vi "Configure SequenceFileView Manager.vi"(8 "error in (no error)":errorcluster, 11 "Auto UI in":refnum<class "Auto UI.lvclass">) -> (0 "error out":errorcluster, 3 "Auto UI out":refnum<class "Auto UI.lvclass">)   [LabVIEW 2023, in "GUI.lvlib" / "Auto UI.lvlib" / "Auto UI.lvclass"]
uses:
  Auto UI.lvclass
  Auto UI.lvclass/Auto UI.ctl
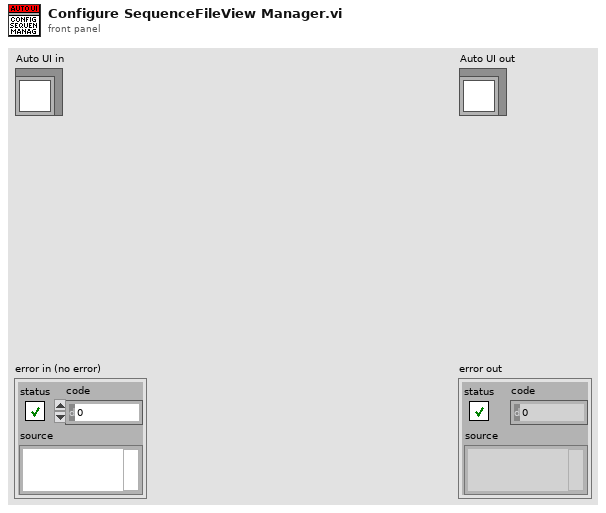
[diagram p1: front panel]
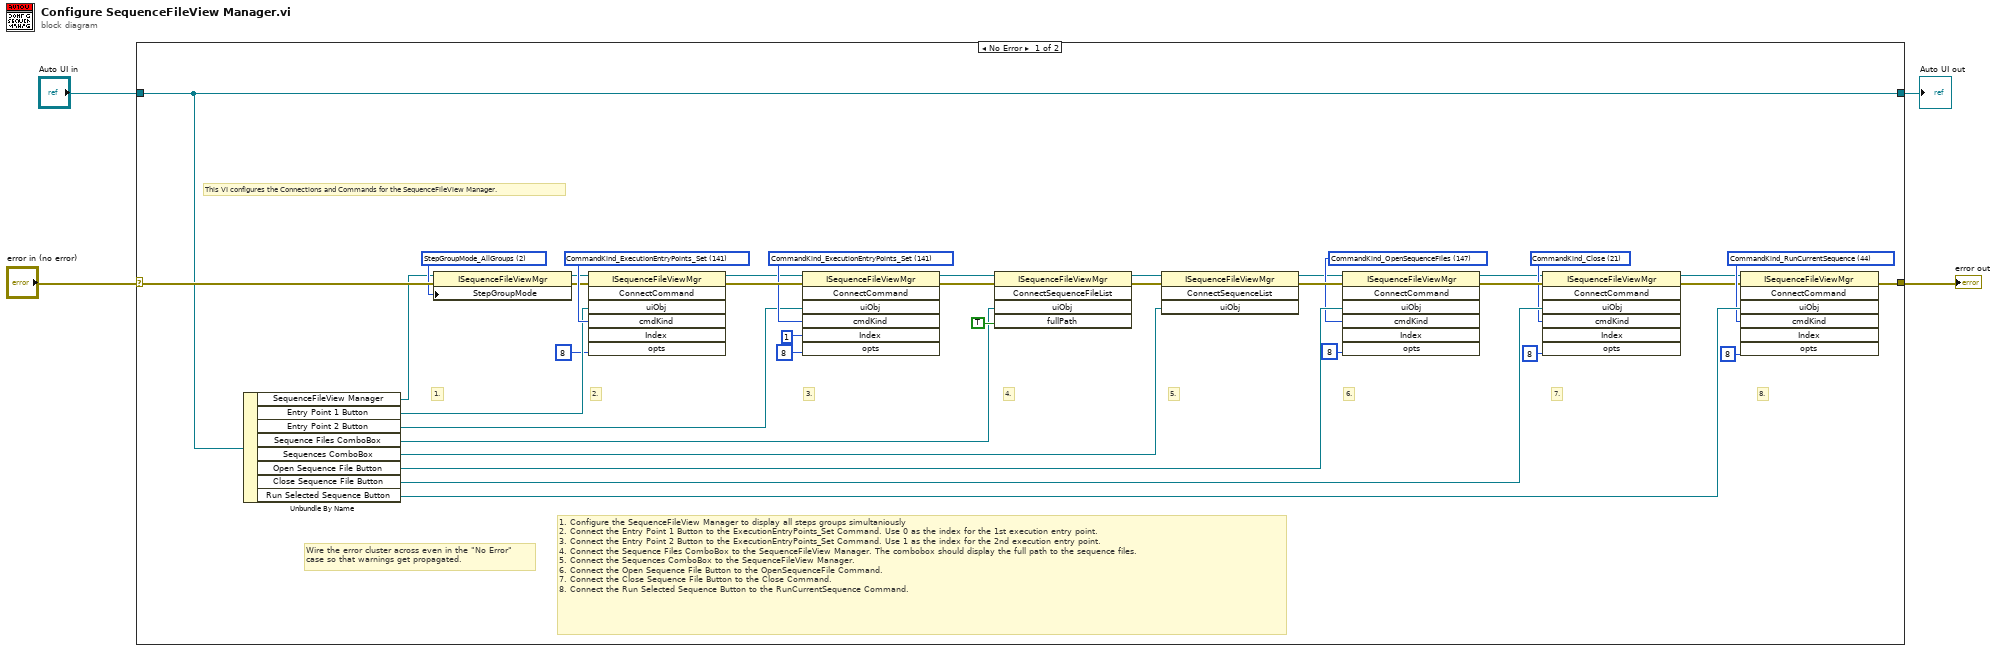
[diagram p0: block diagram]
diagram:
  n1 = case shown="No Error" "error in (no error)" {
    selector: "error in (no error)" -> [w42 w44]
    tunnel: [w41 w44] -> w3
    tunnel: [w5 w43] -> w1
    tunnel: "Auto UI in" -> [w5 w43]
    frame No Error {
      w24 = 2 items=["StepGroupMode_OneGroup"=1, "StepGroupMode_AllGroups"=2] ("StepGroupMode")
      w25 = 147 items=["CommandKind_NotACommand"=0, "CommandKind_Container"=1, "CommandKind_Separator"=2, "CommandKind_Custom"=3, "CommandKind_OpenSequenceFile"=20, "CommandKind_Close"=21, "CommandKind_CloseAll"=22, "CommandKind_CloseCompletedExecutions"=23, "CommandKind_OpenWorkspaceBrowser"=24, "CommandKind_Login"=25, "CommandKind_Logout"=26, "CommandKind_LoginLogout"=27, "CommandKind_UnloadAllModules"=28, "CommandKind_MRUFile"=29, "CommandKind_Exit"=30, "CommandKind_Restart"=40, "CommandKind_RunEntryPoint"=41, "CommandKind_RunEntryPointOnSelectedSteps"=42, "CommandKind_LoopEntryPointOnSelectedSteps"=43, "CommandKind_RunCurrentSequence"=44, "CommandKind_RunSpecificSequence"=45, "CommandKind_RunSelectedSteps"=46, "CommandKind_RunSelectedStepsUsingEntryPointsSubmenu"=47, "CommandKind_LoopOnSelectedSteps"=48, "CommandKind_LoopOnSelectedStepsUsingEntryPointsSubmenu"=49, "CommandKind_BreakOnFirstStep"=50, "CommandKind_BreakOnStepFailure"=51, "CommandKind_BreakOnSequenceFailure"=52, "CommandKind_TracingEnabled"=53, "CommandKind_ToggleBreakpoint"=60, "CommandKind_SetRunModeSubmenu"=61, "CommandKind_RunModeForcePass"=62, "CommandKind_RunModeForceFail"=63, "CommandKind_RunModeSkip"=64, "CommandKind_RunModeNormal"=65, "CommandKind_Resume"=66, "CommandKind_StepInto"=67, "CommandKind_StepOver"=68, "CommandKind_StepOut"=69, "CommandKind_SetNextStep"=70, "CommandKind_Break"=71, "CommandKind_BreakResume"=72, "CommandKind_Terminate"=73, "CommandKind_TerminateRestart"=74, "CommandKind_Abort"=75, "CommandKind_BreakAll"=76, "CommandKind_TerminateAll"=77, "CommandKind_AbortAll"=78, "CommandKind_ResumeAll"=79, "CommandKind_DisplayBreakpointsAndWatchExpressions"=80, "CommandKind_DisplayBreakpointSettings"=81, "CommandKind_BreakpointSubmenu"=85, "CommandKind_ConfigureAdapters"=90, "CommandKind_ConfigureStationOptions"=91, "CommandKind_ConfigureSearchDirectories"=92, "CommandKind_ConfigureExternalViewers"=93, "CommandKind_ToolItem"=100, "CommandKind_CustomizeTools"=101, "CommandKind_ExecutionEntryPointInsertionMarker"=110, "CommandKind_ExecutionEntryPointDefaultMenuInsertionMarker"=111, "CommandKind_ConfigurationEntryPointInsertionMarker"=112, "CommandKind_ConfigurationEntryPointDefaultMenuInsertionMarker"=113, "CommandKind_DefaultFileMenu_Set"=120, "CommandKind_DefaultExecuteMenu_Set"=121, "CommandKind_DefaultDebugMenu_Set"=123, "CommandKind_DefaultConfigureMenu_Set"=124, "CommandKind_DefaultToolsMenu_Set"=125, "CommandKind_DefaultSequenceViewContextMenu_Set"=126, "CommandKind_DefaultListBarContextMenu_Set"=127, "CommandKind_MRUFiles_Set"=140, "CommandKind_ExecutionEntryPoints_Set"=141, "CommandKind_RunSequences_Set"=142, "CommandKind_RunSelectedStepsUsingEntryPoints_Set"=143, "CommandKind_LoopOnSelectedStepsUsingEntryPoints_Set"=144, "CommandKind_ConfigurationEntryPoints_Set"=145, "CommandKind_Tools_Set"=146, "CommandKind_OpenSequenceFiles"=147] ("cmdKind")
      w26 = 44 items=["CommandKind_NotACommand"=0, "CommandKind_Container"=1, "CommandKind_Separator"=2, "CommandKind_Custom"=3, "CommandKind_OpenSequenceFile"=20, "CommandKind_Close"=21, "CommandKind_CloseAll"=22, "CommandKind_CloseCompletedExecutions"=23, "CommandKind_OpenWorkspaceBrowser"=24, "CommandKind_Login"=25, "CommandKind_Logout"=26, "CommandKind_LoginLogout"=27, "CommandKind_UnloadAllModules"=28, "CommandKind_MRUFile"=29, "CommandKind_Exit"=30, "CommandKind_Restart"=40, "CommandKind_RunEntryPoint"=41, "CommandKind_RunEntryPointOnSelectedSteps"=42, "CommandKind_LoopEntryPointOnSelectedSteps"=43, "CommandKind_RunCurrentSequence"=44, "CommandKind_RunSpecificSequence"=45, "CommandKind_RunSelectedSteps"=46, "CommandKind_RunSelectedStepsUsingEntryPointsSubmenu"=47, "CommandKind_LoopOnSelectedSteps"=48, "CommandKind_LoopOnSelectedStepsUsingEntryPointsSubmenu"=49, "CommandKind_BreakOnFirstStep"=50, "CommandKind_BreakOnStepFailure"=51, "CommandKind_BreakOnSequenceFailure"=52, "CommandKind_TracingEnabled"=53, "CommandKind_ToggleBreakpoint"=60, "CommandKind_SetRunModeSubmenu"=61, "CommandKind_RunModeForcePass"=62, "CommandKind_RunModeForceFail"=63, "CommandKind_RunModeSkip"=64, "CommandKind_RunModeNormal"=65, "CommandKind_Resume"=66, "CommandKind_StepInto"=67, "CommandKind_StepOver"=68, "CommandKind_StepOut"=69, "CommandKind_SetNextStep"=70, "CommandKind_Break"=71, "CommandKind_BreakResume"=72, "CommandKind_Terminate"=73, "CommandKind_TerminateRestart"=74, "CommandKind_Abort"=75, "CommandKind_BreakAll"=76, "CommandKind_TerminateAll"=77, "CommandKind_AbortAll"=78, "CommandKind_ResumeAll"=79, "CommandKind_DisplayBreakpointsAndWatchExpressions"=80, "CommandKind_DisplayBreakpointSettings"=81, "CommandKind_BreakpointSubmenu"=85, "CommandKind_ConfigureAdapters"=90, "CommandKind_ConfigureStationOptions"=91, "CommandKind_ConfigureSearchDirectories"=92, "CommandKind_ConfigureExternalViewers"=93, "CommandKind_ToolItem"=100, "CommandKind_CustomizeTools"=101, "CommandKind_ExecutionEntryPointInsertionMarker"=110, "CommandKind_ExecutionEntryPointDefaultMenuInsertionMarker"=111, "CommandKind_ConfigurationEntryPointInsertionMarker"=112, "CommandKind_ConfigurationEntryPointDefaultMenuInsertionMarker"=113, "CommandKind_DefaultFileMenu_Set"=120, "CommandKind_DefaultExecuteMenu_Set"=121, "CommandKind_DefaultDebugMenu_Set"=123, "CommandKind_DefaultConfigureMenu_Set"=124, "CommandKind_DefaultToolsMenu_Set"=125, "CommandKind_DefaultSequenceViewContextMenu_Set"=126, "CommandKind_DefaultListBarContextMenu_Set"=127, "CommandKind_MRUFiles_Set"=140, "CommandKind_ExecutionEntryPoints_Set"=141, "CommandKind_RunSequences_Set"=142, "CommandKind_RunSelectedStepsUsingEntryPoints_Set"=143, "CommandKind_LoopOnSelectedStepsUsingEntryPoints_Set"=144, "CommandKind_ConfigurationEntryPoints_Set"=145, "CommandKind_Tools_Set"=146] ("cmdKind")
      w27 = 141 items=["CommandKind_NotACommand"=0, "CommandKind_Container"=1, "CommandKind_Separator"=2, "CommandKind_Custom"=3, "CommandKind_OpenSequenceFile"=20, "CommandKind_Close"=21, "CommandKind_CloseAll"=22, "CommandKind_CloseCompletedExecutions"=23, "CommandKind_OpenWorkspaceBrowser"=24, "CommandKind_Login"=25, "CommandKind_Logout"=26, "CommandKind_LoginLogout"=27, "CommandKind_UnloadAllModules"=28, "CommandKind_MRUFile"=29, "CommandKind_Exit"=30, "CommandKind_Restart"=40, "CommandKind_RunEntryPoint"=41, "CommandKind_RunEntryPointOnSelectedSteps"=42, "CommandKind_LoopEntryPointOnSelectedSteps"=43, "CommandKind_RunCurrentSequence"=44, "CommandKind_RunSpecificSequence"=45, "CommandKind_RunSelectedSteps"=46, "CommandKind_RunSelectedStepsUsingEntryPointsSubmenu"=47, "CommandKind_LoopOnSelectedSteps"=48, "CommandKind_LoopOnSelectedStepsUsingEntryPointsSubmenu"=49, "CommandKind_BreakOnFirstStep"=50, "CommandKind_BreakOnStepFailure"=51, "CommandKind_BreakOnSequenceFailure"=52, "CommandKind_TracingEnabled"=53, "CommandKind_ToggleBreakpoint"=60, "CommandKind_SetRunModeSubmenu"=61, "CommandKind_RunModeForcePass"=62, "CommandKind_RunModeForceFail"=63, "CommandKind_RunModeSkip"=64, "CommandKind_RunModeNormal"=65, "CommandKind_Resume"=66, "CommandKind_StepInto"=67, "CommandKind_StepOver"=68, "CommandKind_StepOut"=69, "CommandKind_SetNextStep"=70, "CommandKind_Break"=71, "CommandKind_BreakResume"=72, "CommandKind_Terminate"=73, "CommandKind_TerminateRestart"=74, "CommandKind_Abort"=75, "CommandKind_BreakAll"=76, "CommandKind_TerminateAll"=77, "CommandKind_AbortAll"=78, "CommandKind_ResumeAll"=79, "CommandKind_DisplayBreakpointsAndWatchExpressions"=80, "CommandKind_DisplayBreakpointSettings"=81, "CommandKind_BreakpointSubmenu"=85, "CommandKind_ConfigureAdapters"=90, "CommandKind_ConfigureStationOptions"=91, "CommandKind_ConfigureSearchDirectories"=92, "CommandKind_ConfigureExternalViewers"=93, "CommandKind_ToolItem"=100, "CommandKind_CustomizeTools"=101, "CommandKind_ExecutionEntryPointInsertionMarker"=110, "CommandKind_ExecutionEntryPointDefaultMenuInsertionMarker"=111, "CommandKind_ConfigurationEntryPointInsertionMarker"=112, "CommandKind_ConfigurationEntryPointDefaultMenuInsertionMarker"=113, "CommandKind_DefaultFileMenu_Set"=120, "CommandKind_DefaultExecuteMenu_Set"=121, "CommandKind_DefaultDebugMenu_Set"=123, "CommandKind_DefaultConfigureMenu_Set"=124, "CommandKind_DefaultToolsMenu_Set"=125, "CommandKind_DefaultSequenceViewContextMenu_Set"=126, "CommandKind_DefaultListBarContextMenu_Set"=127, "CommandKind_MRUFiles_Set"=140, "CommandKind_ExecutionEntryPoints_Set"=141, "CommandKind_RunSequences_Set"=142, "CommandKind_RunSelectedStepsUsingEntryPoints_Set"=143, "CommandKind_LoopOnSelectedStepsUsingEntryPoints_Set"=144, "CommandKind_ConfigurationEntryPoints_Set"=145, "CommandKind_Tools_Set"=146] ("cmdKind")
      w28 = 141 items=["CommandKind_NotACommand"=0, "CommandKind_Container"=1, "CommandKind_Separator"=2, "CommandKind_Custom"=3, "CommandKind_OpenSequenceFile"=20, "CommandKind_Close"=21, "CommandKind_CloseAll"=22, "CommandKind_CloseCompletedExecutions"=23, "CommandKind_OpenWorkspaceBrowser"=24, "CommandKind_Login"=25, "CommandKind_Logout"=26, "CommandKind_LoginLogout"=27, "CommandKind_UnloadAllModules"=28, "CommandKind_MRUFile"=29, "CommandKind_Exit"=30, "CommandKind_Restart"=40, "CommandKind_RunEntryPoint"=41, "CommandKind_RunEntryPointOnSelectedSteps"=42, "CommandKind_LoopEntryPointOnSelectedSteps"=43, "CommandKind_RunCurrentSequence"=44, "CommandKind_RunSpecificSequence"=45, "CommandKind_RunSelectedSteps"=46, "CommandKind_RunSelectedStepsUsingEntryPointsSubmenu"=47, "CommandKind_LoopOnSelectedSteps"=48, "CommandKind_LoopOnSelectedStepsUsingEntryPointsSubmenu"=49, "CommandKind_BreakOnFirstStep"=50, "CommandKind_BreakOnStepFailure"=51, "CommandKind_BreakOnSequenceFailure"=52, "CommandKind_TracingEnabled"=53, "CommandKind_ToggleBreakpoint"=60, "CommandKind_SetRunModeSubmenu"=61, "CommandKind_RunModeForcePass"=62, "CommandKind_RunModeForceFail"=63, "CommandKind_RunModeSkip"=64, "CommandKind_RunModeNormal"=65, "CommandKind_Resume"=66, "CommandKind_StepInto"=67, "CommandKind_StepOver"=68, "CommandKind_StepOut"=69, "CommandKind_SetNextStep"=70, "CommandKind_Break"=71, "CommandKind_BreakResume"=72, "CommandKind_Terminate"=73, "CommandKind_TerminateRestart"=74, "CommandKind_Abort"=75, "CommandKind_BreakAll"=76, "CommandKind_TerminateAll"=77, "CommandKind_AbortAll"=78, "CommandKind_ResumeAll"=79, "CommandKind_DisplayBreakpointsAndWatchExpressions"=80, "CommandKind_DisplayBreakpointSettings"=81, "CommandKind_BreakpointSubmenu"=85, "CommandKind_ConfigureAdapters"=90, "CommandKind_ConfigureStationOptions"=91, "CommandKind_ConfigureSearchDirectories"=92, "CommandKind_ConfigureExternalViewers"=93, "CommandKind_ToolItem"=100, "CommandKind_CustomizeTools"=101, "CommandKind_ExecutionEntryPointInsertionMarker"=110, "CommandKind_ExecutionEntryPointDefaultMenuInsertionMarker"=111, "CommandKind_ConfigurationEntryPointInsertionMarker"=112, "CommandKind_ConfigurationEntryPointDefaultMenuInsertionMarker"=113, "CommandKind_DefaultFileMenu_Set"=120, "CommandKind_DefaultExecuteMenu_Set"=121, "CommandKind_DefaultDebugMenu_Set"=123, "CommandKind_DefaultConfigureMenu_Set"=124, "CommandKind_DefaultToolsMenu_Set"=125, "CommandKind_DefaultSequenceViewContextMenu_Set"=126, "CommandKind_DefaultListBarContextMenu_Set"=127, "CommandKind_MRUFiles_Set"=140, "CommandKind_ExecutionEntryPoints_Set"=141, "CommandKind_RunSequences_Set"=142, "CommandKind_RunSelectedStepsUsingEntryPoints_Set"=143, "CommandKind_LoopOnSelectedStepsUsingEntryPoints_Set"=144, "CommandKind_ConfigurationEntryPoints_Set"=145, "CommandKind_Tools_Set"=146] ("cmdKind")
      w29 = 21 items=["CommandKind_NotACommand"=0, "CommandKind_Container"=1, "CommandKind_Separator"=2, "CommandKind_Custom"=3, "CommandKind_OpenSequenceFile"=20, "CommandKind_Close"=21, "CommandKind_CloseAll"=22, "CommandKind_CloseCompletedExecutions"=23, "CommandKind_OpenWorkspaceBrowser"=24, "CommandKind_Login"=25, "CommandKind_Logout"=26, "CommandKind_LoginLogout"=27, "CommandKind_UnloadAllModules"=28, "CommandKind_MRUFile"=29, "CommandKind_Exit"=30, "CommandKind_Restart"=40, "CommandKind_RunEntryPoint"=41, "CommandKind_RunEntryPointOnSelectedSteps"=42, "CommandKind_LoopEntryPointOnSelectedSteps"=43, "CommandKind_RunCurrentSequence"=44, "CommandKind_RunSpecificSequence"=45, "CommandKind_RunSelectedSteps"=46, "CommandKind_RunSelectedStepsUsingEntryPointsSubmenu"=47, "CommandKind_LoopOnSelectedSteps"=48, "CommandKind_LoopOnSelectedStepsUsingEntryPointsSubmenu"=49, "CommandKind_BreakOnFirstStep"=50, "CommandKind_BreakOnStepFailure"=51, "CommandKind_BreakOnSequenceFailure"=52, "CommandKind_TracingEnabled"=53, "CommandKind_ToggleBreakpoint"=60, "CommandKind_SetRunModeSubmenu"=61, "CommandKind_RunModeForcePass"=62, "CommandKind_RunModeForceFail"=63, "CommandKind_RunModeSkip"=64, "CommandKind_RunModeNormal"=65, "CommandKind_Resume"=66, "CommandKind_StepInto"=67, "CommandKind_StepOver"=68, "CommandKind_StepOut"=69, "CommandKind_SetNextStep"=70, "CommandKind_Break"=71, "CommandKind_BreakResume"=72, "CommandKind_Terminate"=73, "CommandKind_TerminateRestart"=74, "CommandKind_Abort"=75, "CommandKind_BreakAll"=76, "CommandKind_TerminateAll"=77, "CommandKind_AbortAll"=78, "CommandKind_ResumeAll"=79, "CommandKind_DisplayBreakpointsAndWatchExpressions"=80, "CommandKind_DisplayBreakpointSettings"=81, "CommandKind_BreakpointSubmenu"=85, "CommandKind_ConfigureAdapters"=90, "CommandKind_ConfigureStationOptions"=91, "CommandKind_ConfigureSearchDirectories"=92, "CommandKind_ConfigureExternalViewers"=93, "CommandKind_ToolItem"=100, "CommandKind_CustomizeTools"=101, "CommandKind_ExecutionEntryPointInsertionMarker"=110, "CommandKind_ExecutionEntryPointDefaultMenuInsertionMarker"=111, "CommandKind_ConfigurationEntryPointInsertionMarker"=112, "CommandKind_ConfigurationEntryPointDefaultMenuInsertionMarker"=113, "CommandKind_DefaultFileMenu_Set"=120, "CommandKind_DefaultExecuteMenu_Set"=121, "CommandKind_DefaultDebugMenu_Set"=123, "CommandKind_DefaultConfigureMenu_Set"=124, "CommandKind_DefaultToolsMenu_Set"=125, "CommandKind_DefaultSequenceViewContextMenu_Set"=126, "CommandKind_DefaultListBarContextMenu_Set"=127, "CommandKind_MRUFiles_Set"=140, "CommandKind_ExecutionEntryPoints_Set"=141, "CommandKind_RunSequences_Set"=142, "CommandKind_RunSelectedStepsUsingEntryPoints_Set"=143, "CommandKind_LoopOnSelectedStepsUsingEntryPoints_Set"=144, "CommandKind_ConfigurationEntryPoints_Set"=145, "CommandKind_Tools_Set"=146] ("cmdKind")
      # "8."
      # "7."
      # "6."
      # "5."
      # "4."
      # "3."
      # "2."
      # "1."
      # "1. Configure the SequenceFileView Manager to display all steps groups simultaniously\n2. Connect the Entry Point 1 Button to the ExecutionEntryPoints_Set Command. Use 0 as the index for the 1st execution entry point.\n3. Connect the Entry Point 2 Button to the ExecutionEntryPoints_Set Command. Use 1 as the index for the 2nd execution entry point.\n4. Connect the Sequence Files ComboBox to the SequenceFileView Manager. The combobox should display the full path to the sequence files.\n5. Connect the Sequences ComboBox to the SequenceFileView Manager.\n6. Connect the Open Sequence File Button to the OpenSequenceFile Command.\n7. Connect the Close Sequence File Button to the Close Command.\n8. Connect the Run Selected Sequence Button to the RunCurrentSequence Command."
      # "This VI configures the Connections and Commands for the SequenceFileView Manager."
      # "Wire the error cluster across even in the \"No Error\"\ncase so that warnings get propagated."
      n2 = Unbundle By Name(w5) -> ("SequenceFileView Manager"=w13:refnum<k7>, "Entry Point 1 Button"=w12:refnum<k7>, "Entry Point 2 Button"=w11:refnum<k7>, "Sequence Files ComboBox"=w34:refnum<k7>, "Sequences ComboBox"=w33:refnum<k7>, "Open Sequence File Button"=w30:refnum<k7>, "Close Sequence File Button"=w32:refnum<k7>, "Run Selected Sequence Button"=w31:refnum<k7>)
      n3 = property class="ISequenceFileViewMgr"(reference=w13, error in=w42, "StepGroupMode"=w24) -> (reference out=w20:refnum<k7>, error out=w23:errorcluster)
      n4 = invoke class="ISequenceFileViewMgr" method="ConnectCommand"(reference=w20, error in=w23, "uiObj"=w12, "cmdKind"=w28, "opts"=8) -> (reference out=w19:refnum<k7>, error out=w40:errorcluster)  [unwired: 2 in, 5 out]
      n5 = invoke class="ISequenceFileViewMgr" method="ConnectCommand"(reference=w19, error in=w40, "uiObj"=w11, "cmdKind"=w27, "Index"=1, "opts"=8) -> (reference out=w18:refnum<k7>, error out=w22:errorcluster)  [unwired: 1 in, 5 out]
      n6 = invoke class="ISequenceFileViewMgr" method="ConnectSequenceFileList"(reference=w18, error in=w22, "uiObj"=w34, "fullPath"=TRUE) -> (reference out=w17:refnum<k7>, error out=w37:errorcluster)  [unwired: 1 in, 3 out]
      n7 = invoke class="ISequenceFileViewMgr" method="ConnectSequenceList"(reference=w17, error in=w37, "uiObj"=w33) -> (reference out=w16:refnum<k7>, error out=w38:errorcluster)  [unwired: 1 in, 2 out]
      n8 = invoke class="ISequenceFileViewMgr" method="ConnectCommand"(reference=w16, error in=w38, "uiObj"=w30, "cmdKind"=w25, "opts"=8) -> (reference out=w15:refnum<k7>, error out=w39:errorcluster)  [unwired: 2 in, 5 out]
      n9 = invoke class="ISequenceFileViewMgr" method="ConnectCommand"(reference=w15, error in=w39, "uiObj"=w32, "cmdKind"=w29, "opts"=8) -> (reference out=w14:refnum<k7>, error out=w21:errorcluster)  [unwired: 2 in, 5 out]
      n10 = invoke class="ISequenceFileViewMgr" method="ConnectCommand"(reference=w14, error in=w21, "uiObj"=w31, "cmdKind"=w26, "opts"=8) -> (error out=w41:errorcluster)  [unwired: 2 in, 6 out]
    }
    frame Error {
    }
  }
  "error out" <- w3
  "Auto UI out" <- w1
